vi "AD5781Init.vi"() -> (3 "timeOut":bool)   [LabVIEW 2014]
uses:
  <vilib>/rvi/eio/common/nirviEmuTemplateMethod_errors.vi
  <vilib>/rvi/Emulation/niFpgaSctlEmulationGetInTimedLoop.vi
  Code/FPGA SPI_Globals.vi
  <vilib>/rvi/Emulation/niFpgaProcessEmulError.vi
  <vilib>/rvi/Emulation/niFpgaGetClockAttributes.vi
  <vilib>/rvi/Emulation/niFpgaEmulationReportErrorSimple.vi
  <vilib>/rvi/Emulation/niFpgaCriticalErrorInLSC.vi
  <vilib>/eio/EIONode/EIONode.xnode
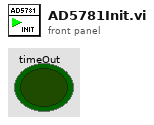
[diagram p1: front panel]
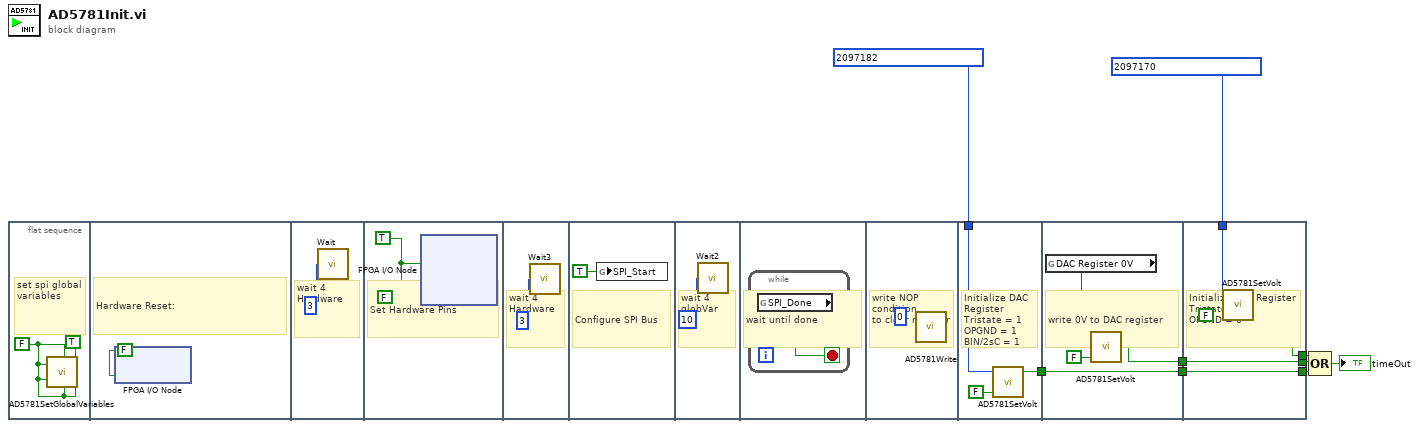
[diagram p0: block diagram]
diagram:
  n1 = flat-sequence {
    tunnel: u32 2097182 ("InitCmd") -> [w23]
    tunnel: [w21] -> w6
    tunnel: w6 -> [w26]
    tunnel: [w26] -> w5
    tunnel: [w25] -> w3
    tunnel: u32 2097170 ("InitCmd") -> [w31]
    tunnel: w5 -> [w30]
    tunnel: [w30] -> w4
    tunnel: w3 -> [w29]
    tunnel: [w29] -> w2
    tunnel: [w28] -> w1
    frame #0 {
      w10 = FALSE ("write DacStateCmdByHost")
      # "set spi global variables"
      n2 = call "AD5781SetGlobalVariables.vi"("write actDACRegister"=w10, "write setDACRegister"=w10, "write DacStateCmdByHost"=w10, "write DacState"=w10, "writeSpiGlobals"=TRUE, "write dac0VRegister"=w10) -> ()  [unwired: 14 in]
    }
    frame #1 {
      # "Hardware Reset:"
      n3 = xnode "FPGA I/O Node"("RESET"=FALSE) -> ()  [unwired: 1 in, 1 out]
    }
    frame #2 {
      # "wait 4\nHardware"
      n4 = call "Wait"("Count(uSec)"=u8 3) -> ()  [unwired: 1 out]
    }
    frame #3 {
      w15 = TRUE ("CLR")
      # "Set Hardware Pins"
      n5 = xnode "FPGA I/O Node"("CLR"=w15, "RESET"=w15, "LDAC"=FALSE ("CLR")) -> ()  [unwired: 3 in, 3 out]
    }
    frame #4 {
      # "wait 4\nHardware"
      n6 = call "Wait3"("Count(uSec)"=u8 3) -> ()  [unwired: 1 out]
    }
    frame #5 {
      # "Configure SPI Bus"
      n7 = global write "FPGA SPI_Globals.vi" "SPI_Start"(TRUE ("SPI_Start")) -> ()
    }
    frame #6 {
      # "wait 4\nglobVar"
      n8 = call "Wait2"("Count(Ticks)"=u8 10 ("Count(uSec)")) -> ()  [unwired: 1 out]
    }
    frame #7 {
      # "wait until done"
      n9 = while {
        stop <- w19 stop-if-true
        n10 = global read "FPGA SPI_Globals.vi" "SPI_Done"() -> (w19:bool)
      }
    }
    frame #8 {
      # "write NOP condition\nto clear register"
      n11 = call "AD5781Write.vi"("U32"=u32 0) -> ()  [unwired: 3 in, 1 out]
    }
    frame #9 {
      # "Initialize DAC Register\nTristate = 1\nOPGND = 1\nBIN/2sC = 1"
      n12 = call "AD5781SetVolt.vi"("Send"=FALSE, "SetVolt"=w23) -> ("timedOut"=w21:bool)  [unwired: 1 in, 2 out]
    }
    frame #10 {
      # "write 0V to DAC register"
      n13 = global read "FPGA SPI_Globals.vi" "DAC Register 0V"() -> (w24:u32)
      n14 = call "AD5781SetVolt.vi"("Send"=FALSE, "SetVolt"=w24) -> ("timedOut"=w25:bool)  [unwired: 1 in, 2 out]
    }
    frame #11 {
      # "Initialize DAC Register\nTristate = 0\nOPGND = 0"
      n15 = call "AD5781SetVolt.vi"("Send"=FALSE, "SetVolt"=w31) -> ("timedOut"=w28:bool)  [unwired: 1 in, 2 out]
    }
  }
  n16 = Compound Arithmetic op=OR(w1, w2, w4) -> (→"timeOut":bool)
